vi "Number of Address Map Elements.vi"(2 "AO in":refnum<class "Analog Output.lvclass">) -> (6 "number of elements":u8)   [LabVIEW 2017, in "Analog IO.lvlib" / "Analog Output.lvclass"]
uses:
  Analog Output.lvclass
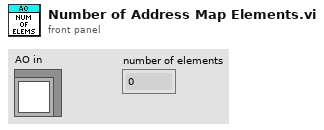
[diagram p1: front panel]
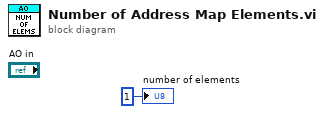
[diagram p0: block diagram]
diagram:
  "number of elements" <- u8 1 ("number of elements")
